vi "Práctica 5 Semáforos.vi"() -> ()   [LabVIEW 2015]
panel:
  out "Verde 2":bool
  out "Rojo 2":bool
  out "Amarillo 2":bool
  out "Contador 2":i32
  in  "stop 2":bool
  out "Estados 3":T1
  out "Estados 2":T1
  in  "stop":bool
  out "Amarillo":bool
  out "Rojo":bool
  out "Verde":bool
  out "Contador":i32
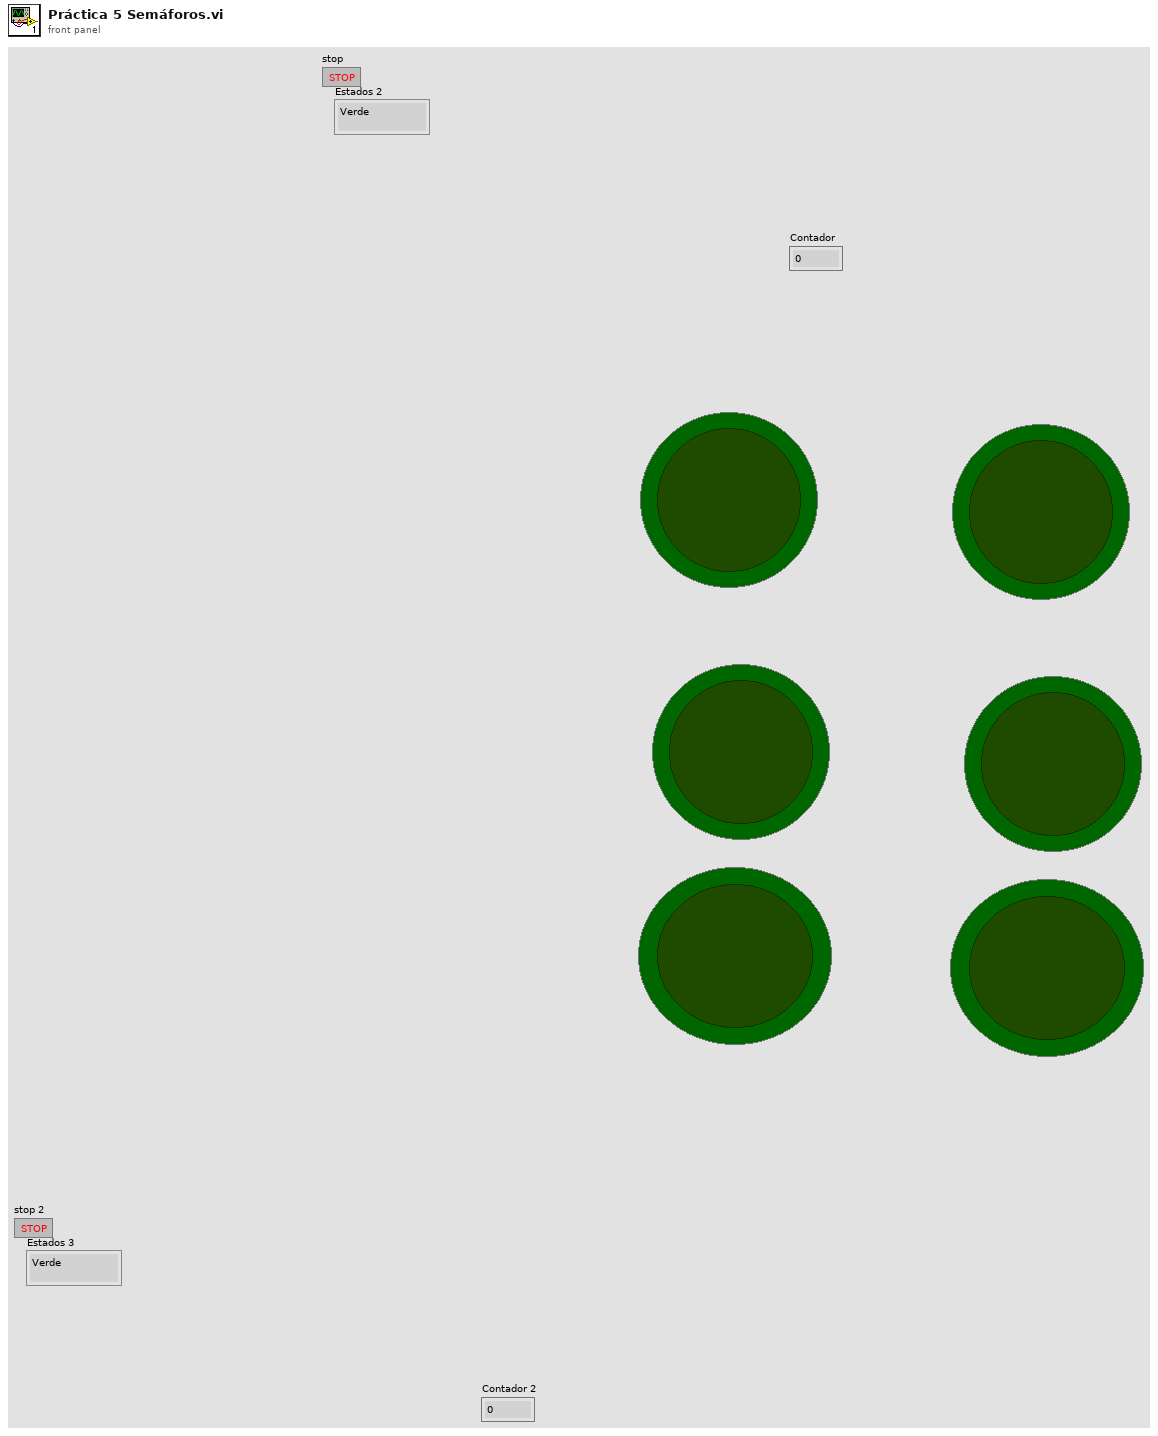
[diagram p1: front panel]
types:
  T1 = typedef "Práctica 3.ctl" = enum16{"Verde", "Parpadeo", "Apagado", "Amarillo", "Rojo"}
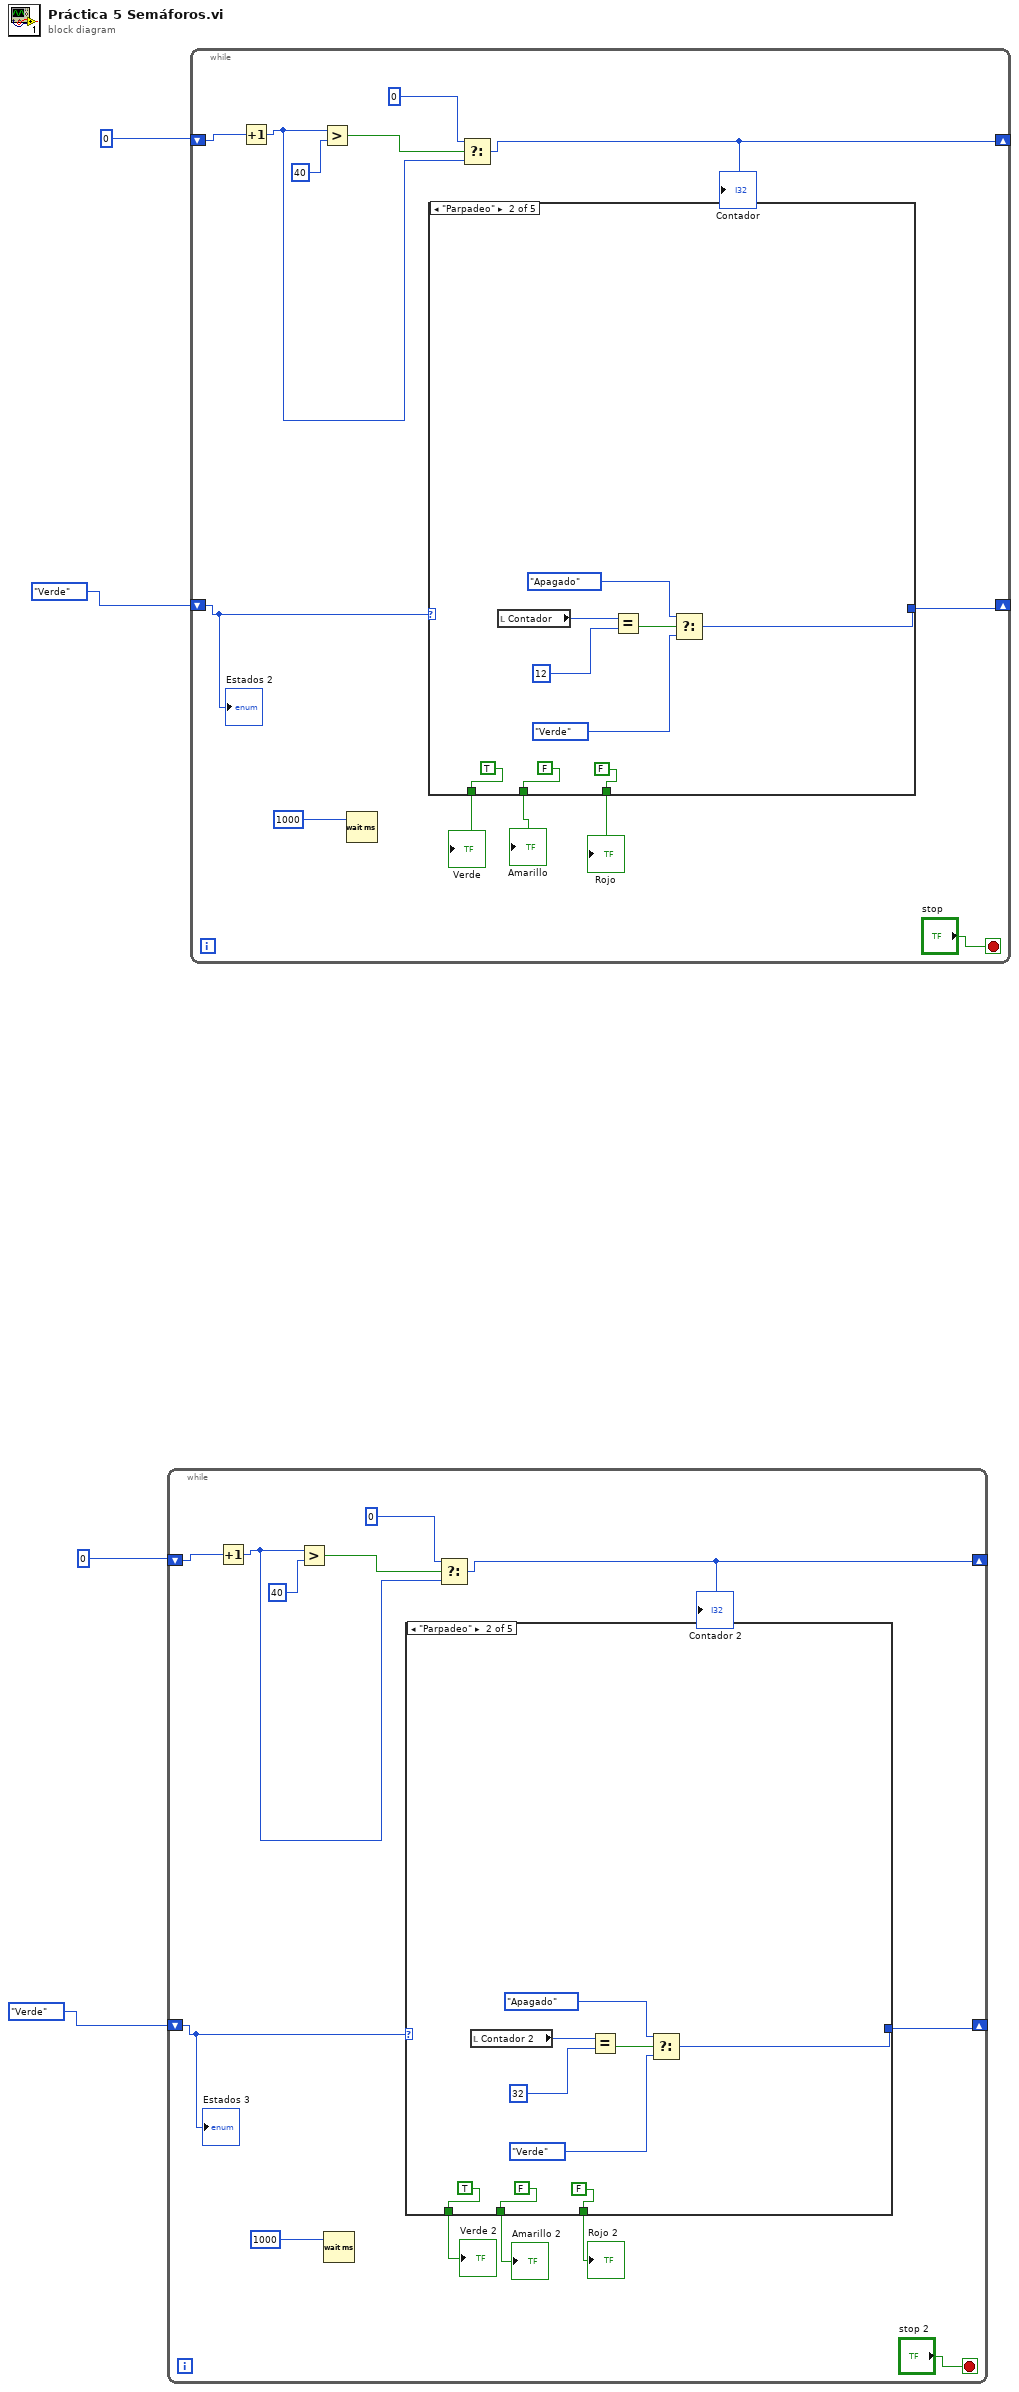
[diagram p0: block diagram]
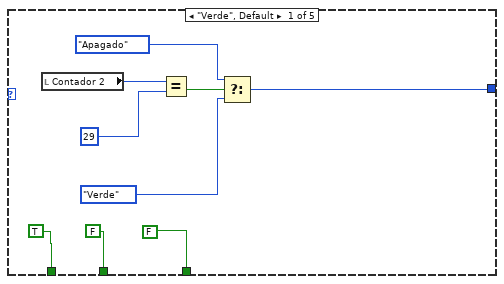
[diagram p2: hidden frame]
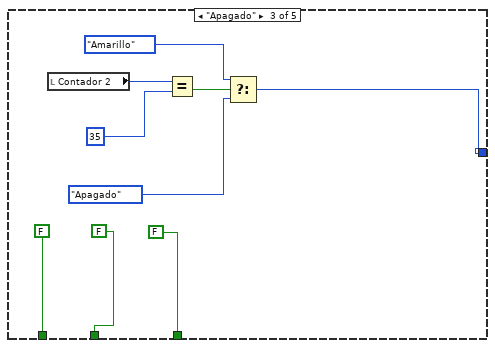
[diagram p3: hidden frame]
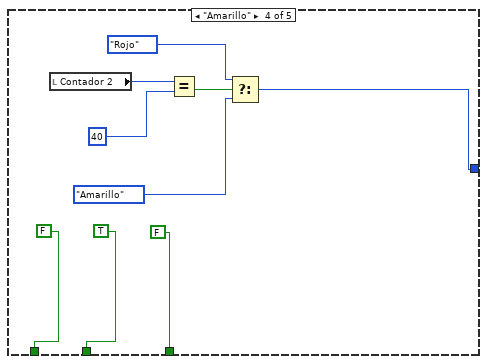
[diagram p4: hidden frame]
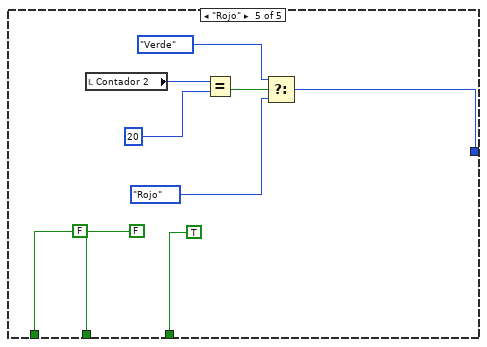
[diagram p5: hidden frame]
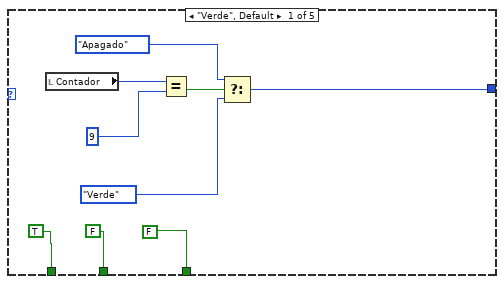
[diagram p6: hidden frame]
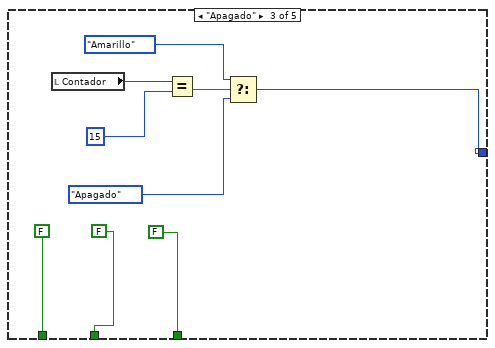
[diagram p7: hidden frame]
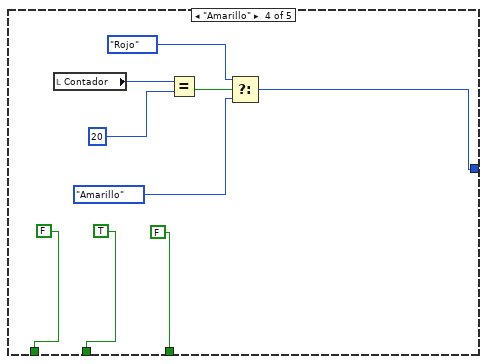
[diagram p8: hidden frame]
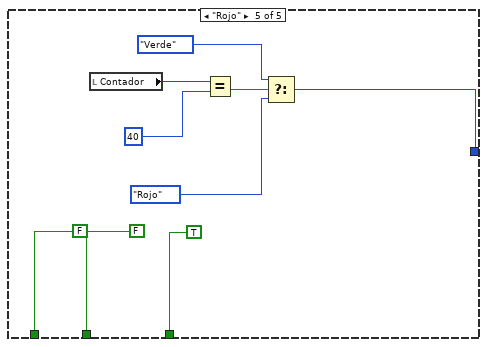
[diagram p9: hidden frame]
diagram:
  n1 = while {
    shift-right: [w12] -> _
    shift-left: 0 -> [w13]
    shift-right: [w10] -> _
    shift-left: Práctica_3."Verde" ("Enum") -> [w8]
    stop <- "stop 2" stop-if-true
    n2 = Increment(x=w13) -> (x+1=w16:i32)
    n3 = Greater?(x=w16, y=40) -> (0:w15:bool)
    n4 = Wait (ms)(milliseconds to wait=1000) -> ()  [unwired: 1 out]
    n5 = case shown="\"Parpadeo\"" w8 {
      tunnel: [w21 w30 w39 w48 w57] -> w10
      tunnel: [TRUE ("Verde") TRUE ("Verde") FALSE ("Verde") FALSE ("Verde") FALSE ("Verde")] -> w7
      tunnel: [FALSE ("Amarillo") FALSE ("Amarillo") FALSE ("Amarillo") TRUE ("Amarillo") FALSE ("Amarillo")] -> w6
      tunnel: [FALSE ("Amarillo") FALSE ("Amarillo") FALSE ("Amarillo") FALSE ("Amarillo") TRUE ("Amarillo")] -> w5
      frame "Verde", Default {
        n6 = local read "Contador 2"() -> (w26:i32)
        n7 = Equal?(x=w26, y=29 ("x")) -> (x = y?=w24:bool)
        n8 = Select(t=Práctica_3."Apagado" ("Enum"), s=w24, f=Práctica_3."Verde" ("Enum")) -> (s? t:f=w21:T1)
      }
      frame "Parpadeo" {
        n9 = local read "Contador 2"() -> (w31:i32)
        n10 = Equal?(x=w31, y=32 ("x")) -> (x = y?=w33:bool)
        n11 = Select(t=Práctica_3."Apagado" ("Enum"), s=w33, f=Práctica_3."Verde" ("Enum")) -> (s? t:f=w30:T1)
      }
      frame "Apagado" {
        n12 = local read "Contador 2"() -> (w40:i32)
        n13 = Equal?(x=w40, y=35 ("x")) -> (x = y?=w42:bool)
        n14 = Select(t=Práctica_3."Amarillo" ("Enum"), s=w42, f=Práctica_3."Apagado" ("Enum")) -> (s? t:f=w39:T1)
      }
      frame "Amarillo" {
        n15 = local read "Contador 2"() -> (w49:i32)
        n16 = Equal?(x=w49, y=40 ("x")) -> (x = y?=w51:bool)
        n17 = Select(t=Práctica_3."Rojo" ("Enum"), s=w51, f=Práctica_3."Amarillo" ("Enum")) -> (s? t:f=w48:T1)
      }
      frame "Rojo" {
        n18 = local read "Contador 2"() -> (w58:i32)
        n19 = Equal?(x=w58, y=20 ("x")) -> (x = y?=w60:bool)
        n20 = Select(t=Práctica_3."Verde" ("Enum"), s=w60, f=Práctica_3."Rojo" ("Enum")) -> (s? t:f=w57:T1)
      }
    }
    "Amarillo 2" <- w6
    "Rojo 2" <- w5
    "Verde 2" <- w7
    n21 = Select(t=0, s=w15, f=w16) -> (s? t:f=w12:i32)
    "Contador 2" <- w12
    "Estados 3" <- w8
  }
  n22 = while {
    shift-right: [w70] -> _
    shift-left: 0 -> [w71]
    shift-right: [w68] -> _
    shift-left: Práctica_3."Verde" ("Enum") -> [w63]
    stop <- "stop" stop-if-true
    n23 = Increment(x=w71) -> (x+1=w74:i32)
    n24 = Greater?(x=w74, y=40) -> (0:w73:bool)
    n25 = Wait (ms)(milliseconds to wait=1000) -> ()  [unwired: 1 out]
    n26 = case shown="\"Parpadeo\"" w63 {
      tunnel: [w79 w88 w97 w106 w115] -> w68
      tunnel: [TRUE ("Verde") TRUE ("Verde") FALSE ("Verde") FALSE ("Verde") FALSE ("Verde")] -> w67
      tunnel: [FALSE ("Amarillo") FALSE ("Amarillo") FALSE ("Amarillo") TRUE ("Amarillo") FALSE ("Amarillo")] -> w66
      tunnel: [FALSE ("Amarillo") FALSE ("Amarillo") FALSE ("Amarillo") FALSE ("Amarillo") TRUE ("Amarillo")] -> w65
      frame "Verde", Default {
        n27 = local read "Contador"() -> (w84:i32)
        n28 = Equal?(x=w84, y=9 ("x")) -> (x = y?=w82:bool)
        n29 = Select(t=Práctica_3."Apagado" ("Enum"), s=w82, f=Práctica_3."Verde" ("Enum")) -> (s? t:f=w79:T1)
      }
      frame "Parpadeo" {
        n30 = local read "Contador"() -> (w89:i32)
        n31 = Equal?(x=w89, y=12 ("x")) -> (x = y?=w91:bool)
        n32 = Select(t=Práctica_3."Apagado" ("Enum"), s=w91, f=Práctica_3."Verde" ("Enum")) -> (s? t:f=w88:T1)
      }
      frame "Apagado" {
        n33 = local read "Contador"() -> (w98:i32)
        n34 = Equal?(x=w98, y=15 ("x")) -> (x = y?=w100:bool)
        n35 = Select(t=Práctica_3."Amarillo" ("Enum"), s=w100, f=Práctica_3."Apagado" ("Enum")) -> (s? t:f=w97:T1)
      }
      frame "Amarillo" {
        n36 = local read "Contador"() -> (w107:i32)
        n37 = Equal?(x=w107, y=20 ("x")) -> (x = y?=w109:bool)
        n38 = Select(t=Práctica_3."Rojo" ("Enum"), s=w109, f=Práctica_3."Amarillo" ("Enum")) -> (s? t:f=w106:T1)
      }
      frame "Rojo" {
        n39 = local read "Contador"() -> (w116:i32)
        n40 = Equal?(x=w116, y=40 ("x")) -> (x = y?=w118:bool)
        n41 = Select(t=Práctica_3."Verde" ("Enum"), s=w118, f=Práctica_3."Rojo" ("Enum")) -> (s? t:f=w115:T1)
      }
    }
    "Rojo" <- w65
    "Verde" <- w67
    "Amarillo" <- w66
    n42 = Select(t=0, s=w73, f=w74) -> (s? t:f=w70:i32)
    "Contador" <- w70
    "Estados 2" <- w63
  }
